vi "Determine Warnings(Modified).vi"() -> ()   [LabVIEW 2014]
panel:
  out "Warning?":bool
  out "Warning Text":string
  in  "Min Temp 2":dbl
  in  "Max Temp":dbl
  in  "Current Temp":dbl
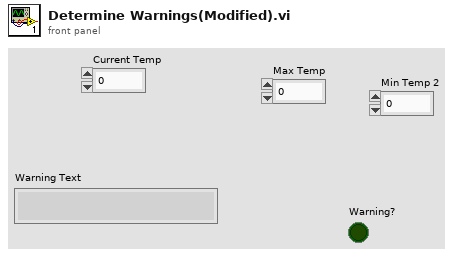
[diagram p1: front panel]
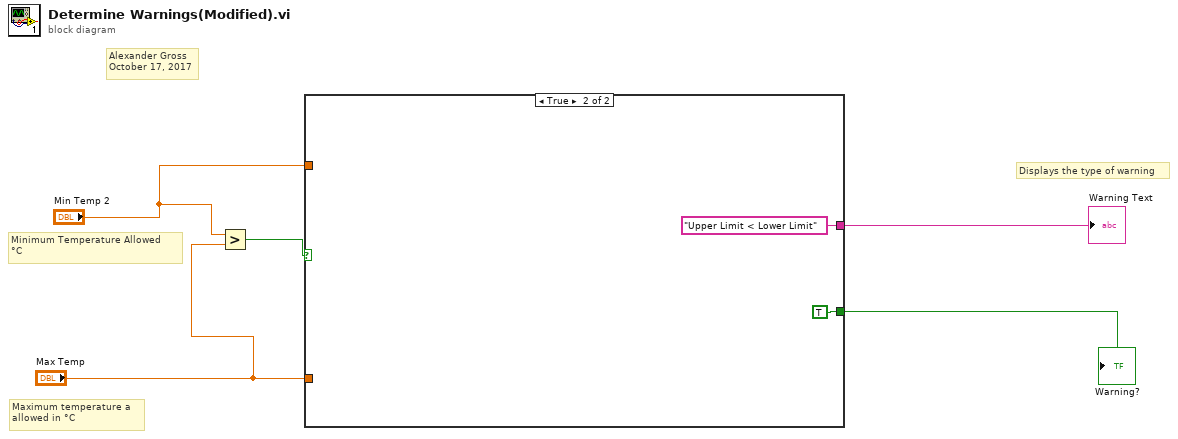
[diagram p0: block diagram]
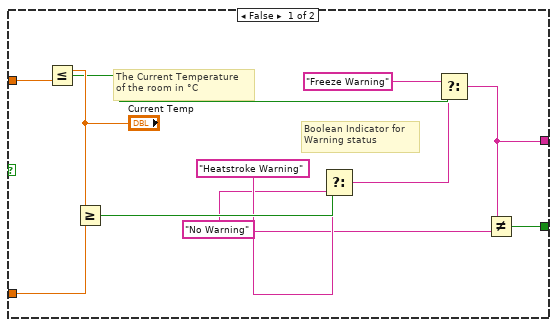
[diagram p2: hidden frame]
diagram:
  # "Alexander Gross\nOctober 17, 2017"
  # "Displays the type of warning"
  # "Minimum Temperature Allowed\n°C"
  # "Maximum temperature a\nallowed in °C"
  n1 = Greater?(x="Min Temp 2", y="Max Temp") -> (0:w1:bool)
  n2 = case shown="True" w1 {
    tunnel: [w9 "Upper Limit < Lower Limit"] -> w5
    tunnel: [w8 TRUE] -> w4
    tunnel: "Min Temp 2" -> [w7 _]
    tunnel: "Max Temp" -> [w6 _]
    frame False {
      w10 = "No Warning"
      # "Boolean Indicator for \nWarning status"
      # "The Current Temperature \nof the room in °C"
      n3 = Less Or Equal?(x="Current Temp", y=w7) -> (x <= y?=w13:bool)
      n4 = Greater Or Equal?(x="Current Temp", y=w6) -> (x >= y?=w15:bool)
      n5 = Select(t="Heatstroke Warning", s=w15, f=w10) -> (s? t:f=w11:string)
      n6 = Select(t="Freeze Warning", s=w13, f=w11) -> (s? t:f=w9:string)
      n7 = Not Equal?(x=w9, y=w10) -> (x != y?=w8:bool)
    }
    frame True {
    }
  }
  "Warning Text" <- w5
  "Warning?" <- w4
